vi "PH_Cam_BaseClass.Open Image.vi"(0 "i ref in":refnum<vi>, 5 "error in":errorcluster) -> (14 "i ref out":refnum<vi>, 19 "error out":errorcluster)   [LabVIEW 2014, in "PH_Cam_BaseClass.lvlib"]
doc: "This VI sets an image to a certain place if it gets the position out of a file stored at the hard drive."
uses:
  PH_Cam_BaseClass.lvlib
  <vilib>/Utility/xml.llb/Read From XML File(array).vi
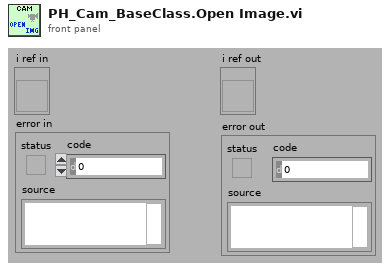
[diagram p1: front panel]
types:
  T1 = typedef "PH_Cam_BaseClass.lvlib/PH_Cam_BaseClass.i attribute.ctl" = cluster{"Gui Refs":T2, "Cam":cluster{"Source Notifier":refnum<notifier>, "Error":errorcluster, "Camera ID":string}, "Images":cluster{"Cam":T3, "Operation":T3, "PSDB":T3}, "Window Image":cluster{"Indicate Image":bool, "Window No.":i32, "Scale Facor":dbl, "Center Cross":bool, "Subtract Backgr":bool, "CoG":bool, "Color Palette":cluster{"Red":u8, "Green":u8, "Blue":u8}[], "Image On":bool}, "Default Prdc Int":i32, "Performance":cluster{"on":bool, "Timestamp Last Frame":i32}, "Histogram":cluster{"on":bool, "Mapping":bool}, "Save Image":cluster{"Save":bool, "File refnum":refnum<file>}, "Setting Service ID":i32, "Screen":cluster{"x-resolution":i16, "y-resolution":i16}, "On":bool, "Constructor finished":bool, "configured":bool}
  T2 = typedef "PH_Cam_BaseClass.lvlib/PH_Cam_BaseClass.GUI Refs.ctl" = cluster{"Frame Rate":refnum<vi>, "Get Frame Rate":refnum<vi>, "Show Image":refnum<vi>, "Get Histogram":refnum<vi>, "Mapping":refnum<vi>, "Histogram":refnum<vi>, "Center Cross":refnum<vi>, "Center of Gravity":refnum<vi>, "Scale Factor [%]":refnum<vi>, "Save Image":refnum<vi>, "Palette":refnum<vi>, "Subtract Background":refnum<vi>, "Cam Error":refnum<vi>, "On":refnum<vi>, "Cam List":refnum<vi>}
  T3 = typedef "IMAQ Image.ctl" = refnum<image>
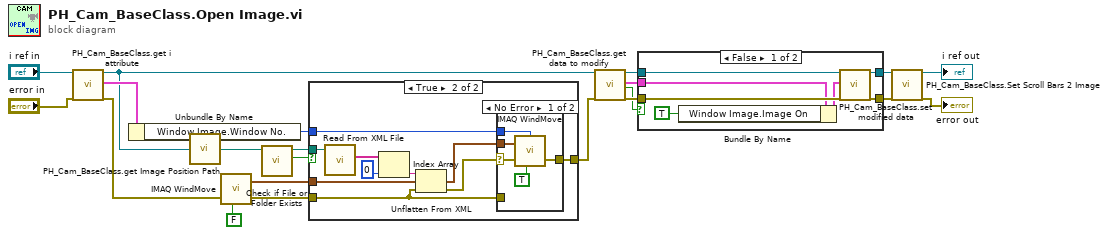
[diagram p0: block diagram]
diagram:
  n1 = call "PH_Cam_BaseClass.get i attribute.vi"("i ref in"="i ref in", "error in (no error)"="error in") -> ("i ref out"=w5:refnum<vi>, "i attribute"=w18:T1, "error out"=w19:errorcluster)  [unwired: 15 in]
  n2 = Unbundle By Name(w18) -> ("Window Image.Window No."=w11:i32)
  n3 = call "PH_Cam_BaseClass.get Image Position Path.vi"("i ref in"=w5) -> ("Image GUI Postion Path"=w13:path)
  n4 = call "IMAQ WindMove"("Get/Set Status? (Set)"=FALSE, "error in (no error)"=w19) -> ("Coordinates (screen)"=w16:cluster{"X Position":i32, "Y Position":i32}, "error out"=w14:errorcluster)  [unwired: 3 in]
  n5 = call <vilib>:"Check if File or Folder Exists.vi"("path"=w13) -> ("file or folder exists?"=w12:bool, "dup path"=w17:path)  [unwired: 8 in, 1 out]
  n6 = case shown="True" w12 {
    tunnel: w16 -> [_ w29]
    tunnel: w17 -> [_ w28]
    tunnel: w14 -> [w22 w23]
    tunnel: w11 -> [_ w26]
    tunnel: [w22 w25] -> w9
    frame False {
    }
    frame True {
      n7 = call-poly <vilib>:"Read From XML File.vi"("XML File Path"=w28) -> ("XML Elements"=w32:string[])  [unwired: 8 in, 2 out]
      n8 = Index Array(array=w32, index=0) -> (element=w30:string)
      n9 = Unflatten From XML(xml string=w30, type=w29, error in (no error)=w23) -> (value=w27:cluster{"X Position":i32, "Y Position":i32}, error out=w24:errorcluster)
      n10 = case shown="No Error" w24 {
        selector: w24 -> [w33 _]
        tunnel: w27 -> [w37 _]
        tunnel: w26 -> [w36 _]
        tunnel: [w35 w38] -> w25
        tunnel: w23 -> [_ w38]
        frame No Error {
          n11 = call "IMAQ WindMove"("Window Number (0...15)"=w36, "Coordinates (screen)"=w37, "Get/Set Status? (Set)"=TRUE, "error in (no error)"=w33) -> ("error out"=w35:errorcluster)  [unwired: 1 in, 1 out]
        }
        frame Error {
        }
      }
    }
  }
  n12 = call "PH_Cam_BaseClass.get data to modify.vi"("i ref in"=w5, "error in (no error)"=w9) -> ("i ref out"=w4:refnum<vi>, "i attribute"=w1:T1, "timed out"=w2:bool, "error out"=w7:errorcluster)  [unwired: 14 in]
  n13 = case shown="False" w2 {
    tunnel: w7 -> [w45 w46]
    tunnel: [w44 w46] -> w6
    tunnel: w4 -> [w43 w47]
    tunnel: [w42 w47] -> w3
    tunnel: w1 -> [w41 _]
    frame False {
      n14 = Bundle By Name(cluster=w41, "Window Image.Image On"=TRUE) -> (w40:T1)
      n15 = call "PH_Cam_BaseClass.set modified data.vi"("i ref in"=w43, "i attribute"=w40, "error in (no error)"=w45) -> ("i ref out"=w42:refnum<vi>, "error out"=w44:errorcluster)  [unwired: 15 in]
    }
    frame True {
    }
  }
  n16 = call "PH_Cam_BaseClass.Set Scroll Bars 2 Image.vi"("i ref in"=w3, "error in (no error)"=w6) -> ("i ref out"=→"i ref out":refnum<vi>, "error out"=→"error out":errorcluster)  [unwired: 16 in]
